vi "Find Workspace.vi"(6 "Pickup_Test_Number":dbl, 8 "Error In":errorcluster, 9 "Assembly Type":string, 10 "Control In":T2={"I-O.lvclass"=refnum, "Gantry"=refnum, "Dispenser"="COM1"}, 11 "Carrier Tray in":refnum<class "Assembly Tray.lvclass">) -> (0 "Error Out":errorcluster, 1 "Workspace":T1, 2 "Control Out":T2={"I-O.lvclass"=refnum, "Gantry"=refnum, "Dispenser"="COM1"}, 3 "Carrier Tray Out":refnum<class "Assembly Tray.lvclass">)   [LabVIEW 2021, in "Assembly Tray.lvclass"]
uses:
  Assembly Tray.lvclass
  C:/Users/HEP/Documents/GitHub/Gantry/UCSB-Gantry-HEP-main/Classes/Workspace/Fixture.lvclass
  Controller/Controllers.ctl
  Controller/I-O/I-O.lvclass
  C:/Program Files (x86)/Aerotech/A3200/LabVIEW/2010/Bin/Aerotech.A3200.dll
  Program Files (x86)/Aerotech/A3200/LabVIEW/2010/Bin/Aerotech.A3200.dll
  Workspace.ctl
  Fixture.lvclass/Fixture.ctl
  Assembly Tray.lvclass/Assembly Tray.ctl
  Read Fixture ID.vi
  Read Position.vi
  Fixture.lvclass
  Controller/Controller.lvclass
panel:
  out "XYZTheta Centers":dbl[][](array[numeric])
  in  "output cluster 2":T1
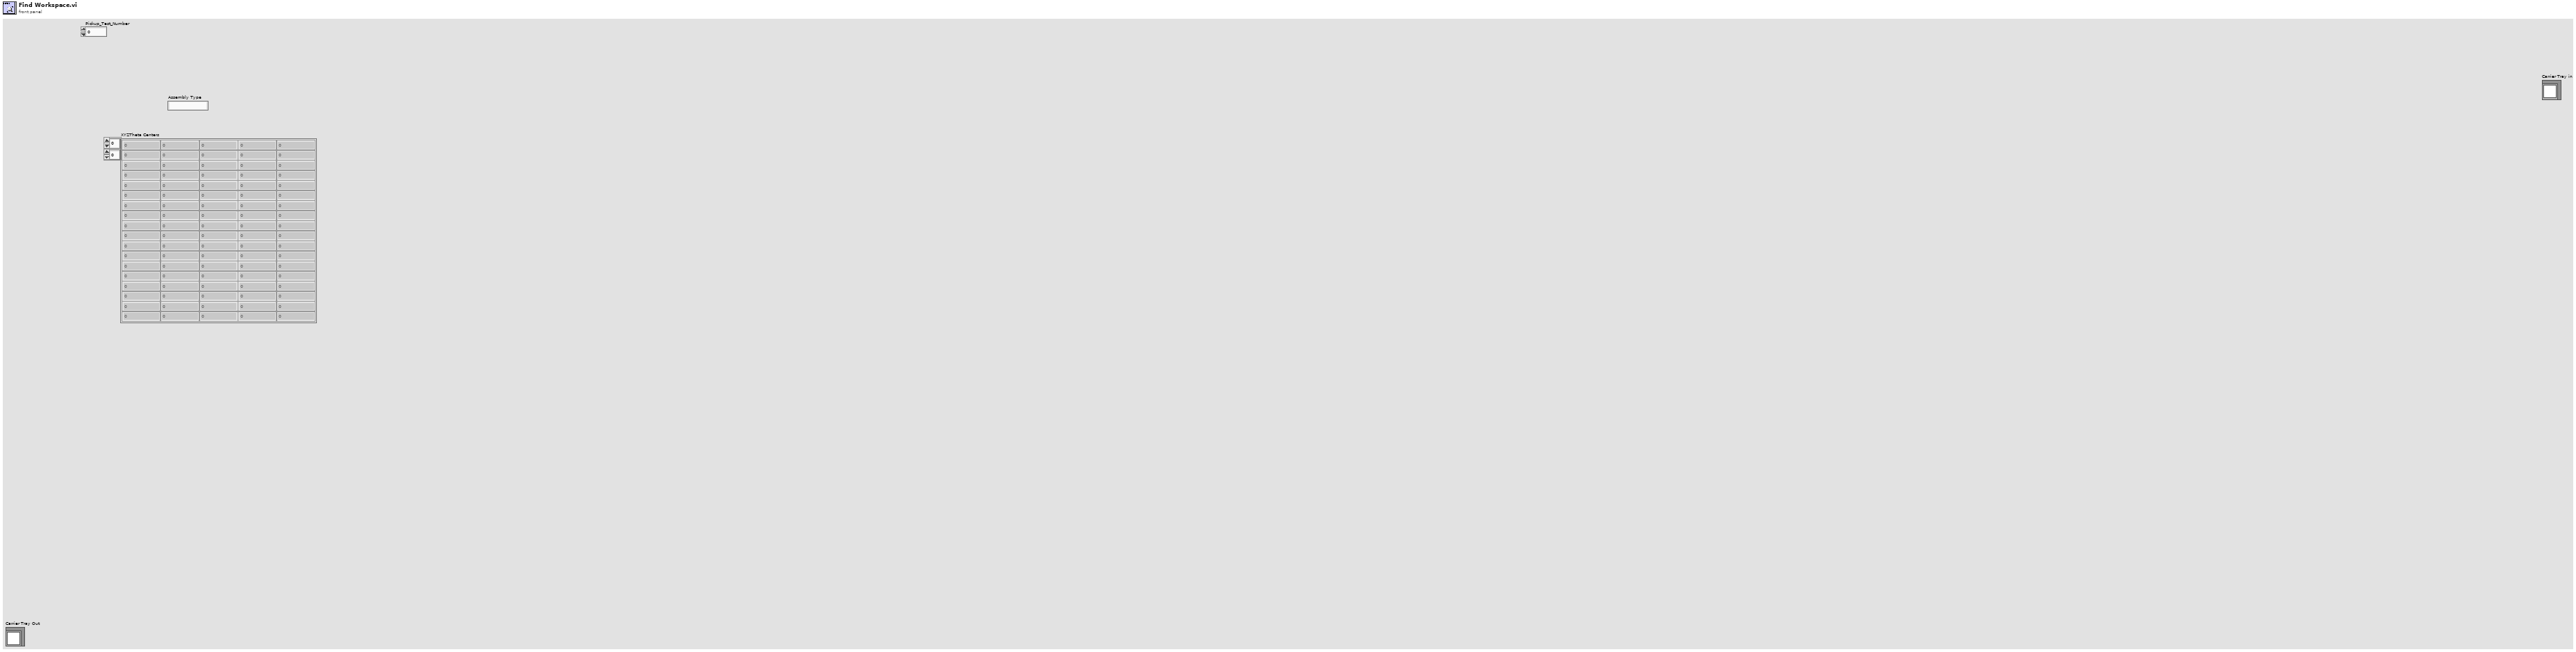
[diagram p1: front panel]
types:
  T1 = typedef "Fixture.lvclass/Workspace.ctl" = cluster{"XYZTheta":dbl[], "Workspace Valve":i32, "Workspace Sensor":i32}
  T2 = typedef "Controller.lvclass/Controllers.ctl" = cluster{"I-O.lvclass":refnum<class "I-O.lvclass">, "Gantry":refnum<k24>, "Dispenser":refnum<visa-resource-name>}
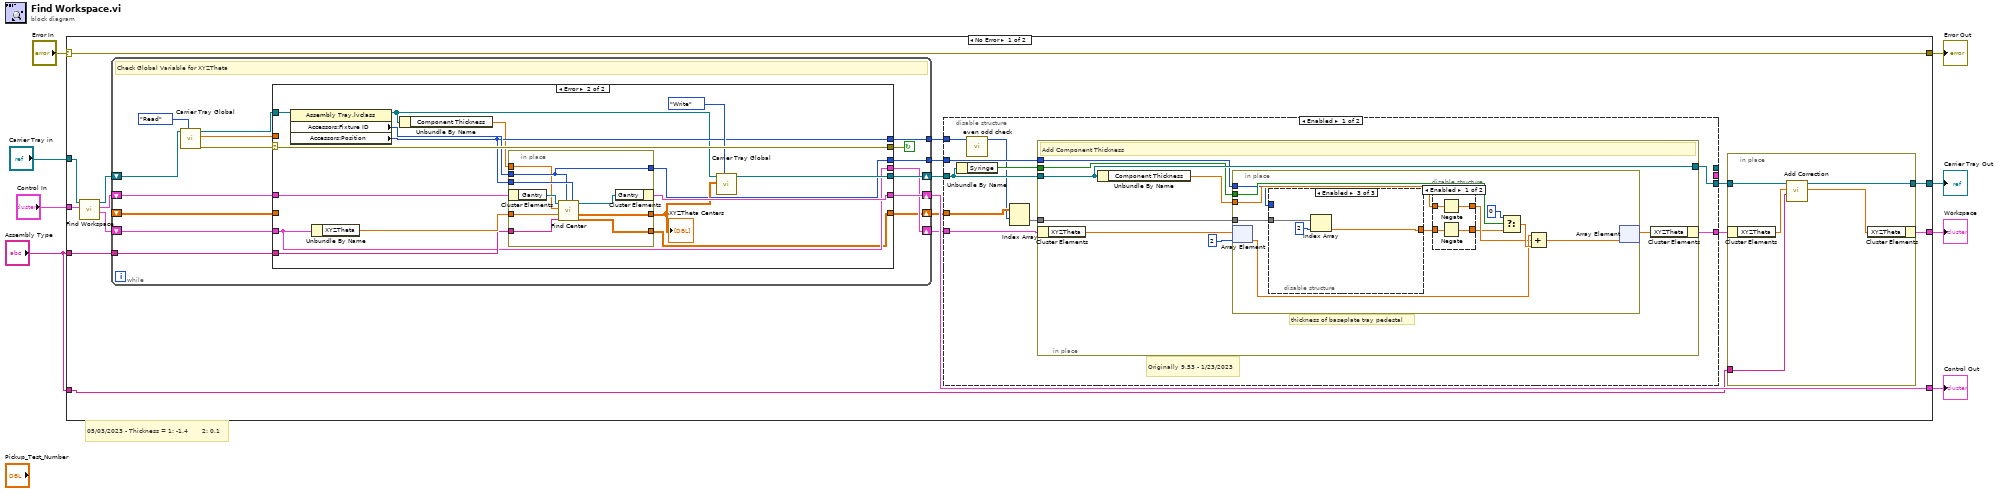
[diagram p0: block diagram]
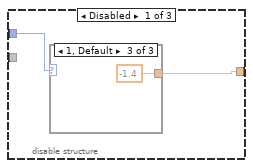
[diagram p2: hidden frame]
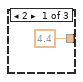
[diagram p3: hidden frame]
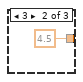
[diagram p4: hidden frame]
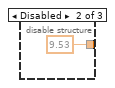
[diagram p5: hidden frame]
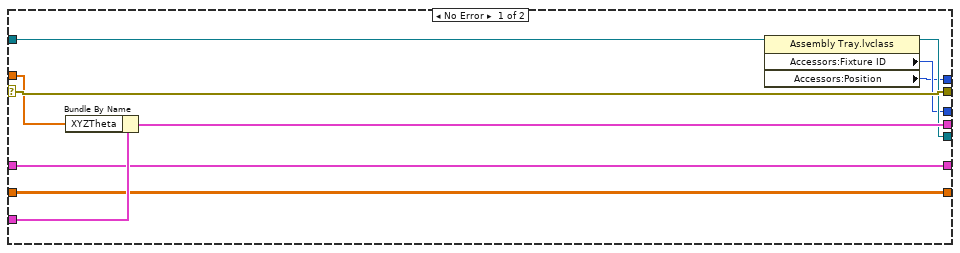
[diagram p8: hidden frame]
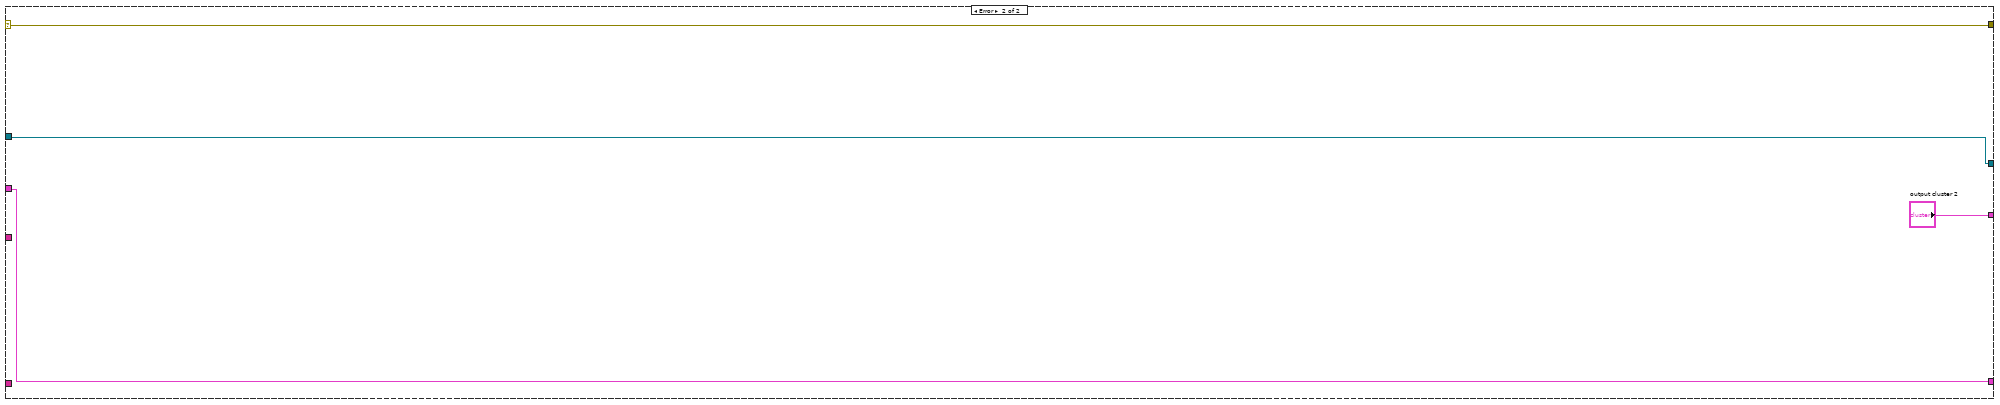
[diagram p9: hidden frame]
diagram:
  # "05/03/2023 - Thickness = 1: -1.4       2: 0.1"
  n1 = case shown="No Error" "Error In" {
    selector: "Error In" -> [w26 w131]
    tunnel: [w26 w131] -> w7
    tunnel: "Control In" -> [w25 w132]
    tunnel: [w23 w132] -> w5
    tunnel: "Carrier Tray in" -> [w24 w129]
    tunnel: [w11 "output cluster 2"] -> w3
    tunnel: [w10 w129] -> w2
    tunnel: "Assembly Type" -> [w17 _]
    tunnel: "Assembly Type" -> [w12 _]
    frame No Error {
      n2 = call-parent "Find Workspace.vi"("Control In"=w25, "Workspace In"=w24) -> (1:"Workspace Out"=w22:T1, "Control Out"=w21:T2, 3:"Workspace Out"=w18:refnum<class "Assembly Tray.lvclass">)  [unwired: 6 in, 1 out]
      n3 = while {
        shift-right: [w86] -> w20
        shift-left: w18 -> [w84]
        shift-right: [w88] -> w23
        shift-left: w21 -> [w89]
        shift-right: [w85] -> w19
        shift-left: w22 -> [w90]
        tunnel: w17 -> [w82]
        tunnel: [w81] -> w16
        shift-right: [w80] -> w15
        shift-left: _ -> [w79]
        tunnel: [w78] -> w9
        stop <- w92 continue-if-true
        # "Check Global Variable for XYZTheta"
        n4 = call "Carrier Tray Global.vi"("Action"=enum16{"Initialize", "Read", "Write"}."Read", "Carrier Tray.lvclass"=w84) -> ("error out"=w83:errorcluster, "XYZTheta out"=w91:dbl[], "Carrier Tray.lvclass 2"=w87:refnum<class "Assembly Tray.lvclass">)  [unwired: 7 in]
        n5 = case shown="Error" w83 {
          selector: w83 -> [w103 w119]
          tunnel: [w103 w119] -> w92
          tunnel: w91 -> [w102 _]
          tunnel: [w101 w108] -> w85
          tunnel: w90 -> [w100 w108]
          tunnel: w89 -> [w99 w114]
          tunnel: [w99 w113] -> w88
          tunnel: w87 -> [w98 w116]
          tunnel: [w97 w118] -> w86
          tunnel: w82 -> [_ w110]
          tunnel: [w96 w109] -> w81
          tunnel: [w95 w107] -> w80
          tunnel: w79 -> [w95 _]
          tunnel: [w94 w106] -> w78
          frame No Error {
            n6 = Bundle By Name(cluster=w100, "XYZTheta"=w102) -> (w101:T1)
            n7 = property class="Assembly Tray.lvclass"(reference=w98) -> (reference out=w97:refnum<class "Assembly Tray.lvclass">, "Accessors:Fixture ID"=w96:i32, "Accessors:Position"=w94:i32)  [unwired: 1 in, 1 out]
          }
          frame Error {
            n8 = property class="Assembly Tray.lvclass"(reference=w116) -> (reference out=w105:refnum<class "Assembly Tray.lvclass">, "Accessors:Fixture ID"=w115:i32, "Accessors:Position"=w106:i32)  [unwired: 1 in, 1 out]
            n9 = Unbundle By Name(w108) -> ("XYZTheta"=w112:dbl[])
            n10 = Unbundle By Name(w105) -> ("Component Thickness"=w104:dbl)
            n11 = in-place {
              in-place-border: w115 -> [w122]
              in-place-border: w112 -> [w126]
              in-place-border: [w125] -> w111
              in-place-border: w110 -> [w124]
              in-place-border: w106 -> [w123]
              in-place-border: [w122] -> w109
              in-place-border: [w121] -> w107
              in-place-border: w104 -> [w120]
              n12 = in-place-cluster #1(w114) -> ("Gantry"=w128:refnum<k24>)
              n13 = call "Find Center.vi"("Position"=w123, "Tray Number"=w122, "Assembly Type"=w124, "XYZTheta"=w126, "component thickness"=w120, "Gantry In"=w128) -> ("Pedestal Heights"=w121:dbl[][], "XYZTheta Centers"=w125:dbl[][], "Gantry Out"=w127:refnum<k24>)  [unwired: 3 in]
              n14 = in-place-cluster #1("Gantry"=w127) -> (w113:T2)
            }
            "XYZTheta Centers" <- w111
            n15 = call "Carrier Tray Global.vi"("Action"=enum16{"Initialize", "Read", "Write"}."Write", "XYZTheta in"=w111, "Carrier Tray.lvclass"=w105) -> ("Carrier Tray.lvclass 2"=w118:refnum<class "Assembly Tray.lvclass">)  [unwired: 6 in, 2 out]
          }
        }
      }
      n16 = disable-structure shown="Enabled" {
        disable-tunnel: [_ w76] -> _
        disable-tunnel: [_ w77] -> _
        disable-tunnel: w20 -> [w41 w76]
        disable-tunnel: w19 -> [w40 w77]
        disable-tunnel: w16 -> [w38 _]
        disable-tunnel: w15 -> [w35 _]
        disable-tunnel: [w37 _] -> w14
        disable-tunnel: [w36 _] -> w13
        disable-tunnel: w9 -> [w32 _]
        frame Enabled {
          # "Originally 9.53 - 1/23/2023"
          n17 = Unbundle By Name(w41) -> ("Syringe"=w39:bool)
          n18 = call "even odd check.vi"("position"=w32) -> ("index"=w33:i32)  [unwired: 10 in]
          n19 = Index Array(array=w35, index (row)=w33) -> (element=w34:dbl[])  [unwired: 1 in]
          n20 = in-place {
            in-place-border: w41 -> [w47]
            in-place-border: [w47] -> w36
            in-place-border: w39 -> [w46]
            in-place-border: w38 -> [w44]
            in-place-border: w34 -> [w42]
            # "thickness of baseplate tray pedestal"
            # "Add Component Thickness"
            n21 = in-place-cluster #2(w40) -> ("XYZTheta"=w45:dbl[])
            n22 = Unbundle By Name(w47) -> ("Component Thickness"=w48:dbl)
            n23 = in-place {
              in-place-border: w48 -> [w55]
              in-place-border: w46 -> [w59]
              in-place-border: w44 -> [w51]
              in-place-border: w42 -> [w50]
              n24 = in-place-array #3(w45, 2) -> (w56:dbl)
              n25 = disable-structure shown="Enabled" {
                disable-tunnel: [w62 9.53 w69] -> w53
                disable-tunnel: w51 -> [w61 _ _]
                disable-tunnel: w50 -> [_ _ w68]
                frame Disabled {
                  n26 = case shown="1, Default" w61 {
                    tunnel: [4.4 4.5 -1.4] -> w62
                    frame 2 {
                    }
                    frame 3 {
                    }
                    frame 1, Default {
                    }
                  }
                }
                frame Disabled {
                }
                frame Enabled {
                  n27 = Index Array(array=w68, index=2) -> (element=w69:dbl)
                }
              }
              n28 = disable-structure shown="Enabled" {
                disable-tunnel: w55 -> [w73 w75]
                disable-tunnel: [w72 w75] -> w54
                disable-tunnel: w53 -> [w71 w74]
                disable-tunnel: [w70 w74] -> w52
                frame Enabled {
                  n29 = Negate(x=w73) -> (-x=w72:dbl)
                  n30 = Negate(x=w71) -> (-x=w70:dbl)
                }
                frame Disabled {
                }
              }
              n31 = Select(t=0, s=w59, f=w52) -> (s? t:f=w57:dbl)
              n32 = Compound Arithmetic op=ADD(w56, w54, w57) -> (w60:dbl)
              n33 = in-place-array #3(w60) -> (w49:dbl[])  [unwired: 1 out]
            }
            n34 = in-place-cluster #2("XYZTheta"=w49) -> (w37:T1)
          }
        }
        frame Disabled {
        }
      }
      n35 = in-place {
        in-place-border: [w31] -> w10
        in-place-border: w13 -> [w30]
        in-place-border: w12 -> [w27]
        n36 = in-place-cluster #4(w14) -> ("XYZTheta"=w29:dbl[])
        n37 = call "Add Correction.vi"("Assembly Type"=w27, "XYZTheta"=w29, "Carrier Tray in"=w30) -> ("XYZTheta Out"=w28:dbl[], "Carrier Tray out"=w31:refnum<class "Assembly Tray.lvclass">)  [unwired: 6 in, 1 out]
        n38 = in-place-cluster #4("XYZTheta"=w28) -> (w11:T1)
      }
    }
    frame Error {
    }
  }
  "Error Out" <- w7
  "Control Out" <- w5
  "Workspace" <- w3
  "Carrier Tray Out" <- w2
